vi "RPM to Fuel Flow.vi"(11 "Requested RPM":dbl=44000.0 min=44000.0 max=135000.0) -> (3 "Fuel Pump Value 1":i32)   [LabVIEW 2017]
panel:
  # "NOTE:\nThere are data entry limits\non this input. These may need\nto be deleted in the future"
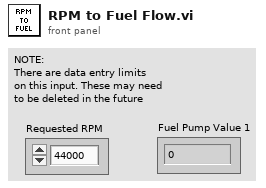
[diagram p1: front panel]
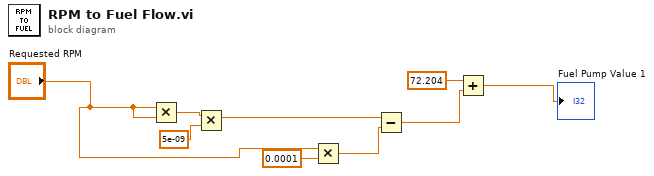
[diagram p0: block diagram]
diagram:
  n1 = Multiply(x="Requested RPM", y="Requested RPM") -> (x*y=w9:dbl)
  n2 = Multiply(x=w9, y=5e-09) -> (x*y=w7:dbl)
  n3 = Multiply(x="Requested RPM", y=0.0001) -> (x*y=w4:dbl)
  n4 = Subtract(x=w7, y=w4) -> (x-y=w3:dbl)
  n5 = Add(x=72.204, y=w3) -> (x+y=→"Fuel Pump Value 1":dbl)
